vi "IO@SetPortName__Parameter.vi"(1 "ParamterIn":string) -> (0 "ParamterOut":string)   [LabVIEW 2020]
panel:
  in  "PortNameNew":string(combo)
  in  "PortSelect":string(combo)
  in  "Confirm":bool
  # "IO@SetPortName $IOOld,$IONew"
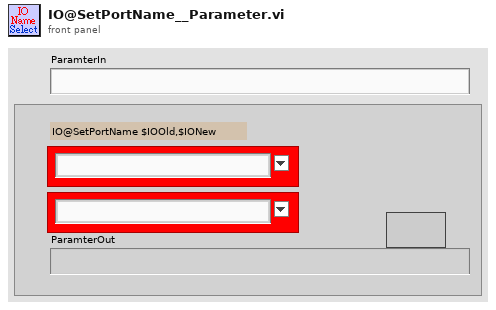
[diagram p1: front panel]
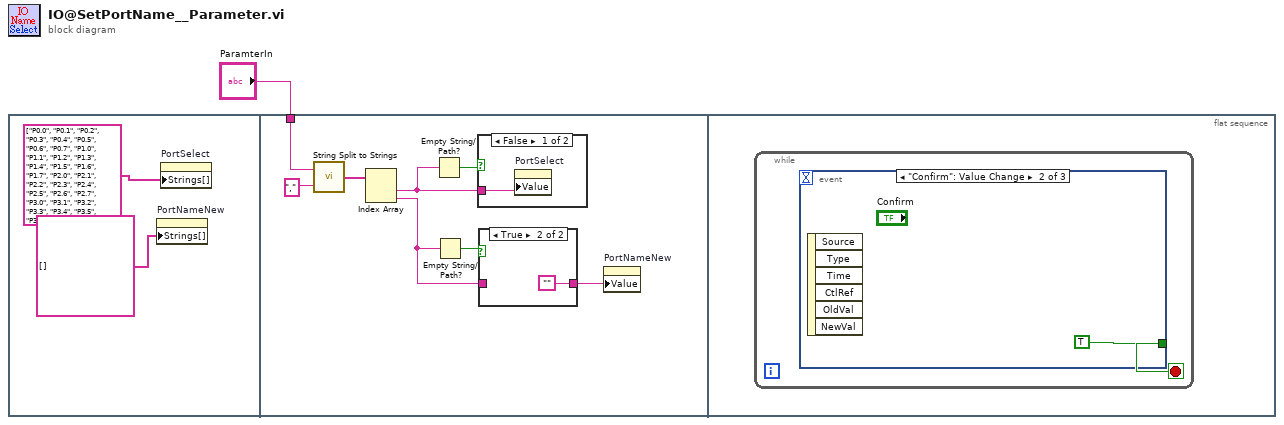
[diagram p0: block diagram]
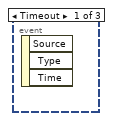
[diagram p4: hidden frame]
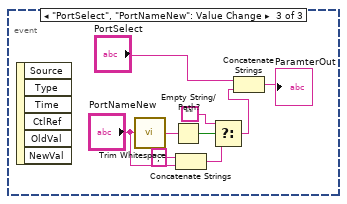
[diagram p5: hidden frame]
diagram:
  n1 = flat-sequence {
    tunnel: "ParamterIn" -> [w9]
    frame #0 {
      n2 = property on="PortNameNew" class="CmbBox"("Strings[]"=string[] [] ("Strings []")) -> ()  [unwired: 2 in, 2 out]
      n3 = property on="PortSelect" class="CmbBox"("Strings[]"=string[] ["P0.0", "P0.1", "P0.2", "P0.3", "P0.4", "P0.5", "P0.6", "P0.7", "P1.0", "P1.1", "P1.2", "P1.3", "P1.4", "P1.5", "P1.6", "P1.7", "P2.0", "P2.1", "P2.2", "P2.3", "P2.4", "P2.5", "P2.6", "P2.7", "P3.0", "P3.1", "P3.2", "P3.3", "P3.4", "P3.5", "P3.6", "P3.7", "P4.0", "P4.1", "P4.2", "P4.3", "P4.4", "P4.5", "P4.6", "P4.7", "P5.0", "P5.1", "P5.2", "P5.3", "P5.4", "P5.5", "P5.6", "P5.7", "P6.0", "P6.1", "P6.2", "P6.3", "P6.4", "P6.5", "P6.6", "P6.7", "P7.0", "P7.1", "P7.2", "P7.3", "P7.4", "P7.5", "P7.6", "P7.7", "P8.0", "P8.1", "P8.2", "P8.3", "P8.4", "P8.5", "P8.6", "P8.7", "P9.0", "P9.1", "P9.2", "P9.3", "P9.4", "P9.5", "P9.6", "P9.7", "P10.0", "P10.1", "P10.2", "P10.3", "P10.4", "P10.5", "P10.6", "P10.7", "P11.0", "P11.1", "P11.2", "P11.3", "P11.4", "P11.5", "P11.6", "P11.7", "P12.0", "P12.1", "P12.2", "P12.3", "P12.4", "P12.5", "P12.6", "P12.7", "P13.0", "P13.1", "P13.2", "P13.3", "P13.4", "P13.5", "P13.6", "P13.7", "P14.0", "P14.1", "P14.2", "P14.3", "P14.4", "P14.5", "P14.6", "P14.7", "P15.0", "P15.1", "P15.2", "P15.3", "P15.4", "P15.5", "P15.6", "P15.7", "P16.0", "P16.1", "P16.2", "P16.3", "P16.4", "P16.5", "P16.6", "P16.7", "P17.0", "P17.1", "P17.2", "P17.3", "P17.4", "P17.5", "P17.6", "P17.7", "P18.0", "P18.1", "P18.2", "P18.3", "P18.4", "P18.5", "P18.6", "P18.7", "P19.0", "P19.1", "P19.2", "P19.3", "P19.4", "P19.5", "P19.6", "P19.7", "P20.0", "P20.1", "P20.2", "P20.3", "P20.4", "P20.5", "P20.6", "P20.7", "P21.0", "P21.1", "P21.2", "P21.3", "P21.4", "P21.5", "P21.6", "P21.7", "P22.0", "P22.1", "P22.2", "P22.3", "P22.4", "P22.5", "P22.6", "P22.7", "P23.0", "P23.1", "P23.2", "P23.3", "P23.4", "P23.5", "P23.6", "P23.7", "P24.0", "P24.1", "P24.2", "P24.3", "P24.4", "P24.5", "P24.6", "P24.7", "P25.0", "P25.1", "P25.2", "P25.3", "P25.4", "P25.5", "P25.6", "P25.7", "P26.0", "P26.1", "P26.2", "P26.3", "P26.4", "P26.5", "P26.6", "P26.7", "P27.0", "P27.1", "P27.2", "P27.3", "P27.4", "P27.5", "P27.6", "P27.7", "P28.0", "P28.1", "P28.2", "P28.3", "P28.4", "P28.5", "P28.6", "P28.7", "P29.0", "P29.1", "P29.2", "P29.3", "P29.4", "P29.5", "P29.6", "P29.7", "P30.0", "P30.1", "P30.2", "P30.3", "P30.4", "P30.5", "P30.6", "P30.7", "P31.0", "P31.1", "P31.2", "P31.3", "P31.4", "P31.5", "P31.6", "P31.7", "P32.0", "P32.1", "P32.2", "P32.3", "P32.4", "P32.5", "P32.6", "P32.7", "P33.0", "P33.1", "P33.2", "P33.3", "P33.4", "P33.5", "P33.6", "P33.7", "P34.0", "P34.1", "P34.2", "P34.3", "P34.4", "P34.5", "P34.6", "P34.7", "P35.0", "P35.1", "P35.2", "P35.3", "P35.4", "P35.5", "P35.6", "P35.7", "P36.0", "P36.1", "P36.2", "P36.3", "P36.4", "P36.5", "P36.6", "P36.7", "P37.0", "P37.1", "P37.2", "P37.3", "P37.4", "P37.5", "P37.6", "P37.7", "P38.0", "P38.1", "P38.2", "P38.3", "P38.4", "P38.5", "P38.6", "P38.7", "P39.0", "P39.1", "P39.2", "P39.3", "P39.4", "P39.5", "P39.6", "P39.7", "P40.0", "P40.1", "P40.2", "P40.3", "P40.4", "P40.5", "P40.6", "P40.7", "P41.0", "P41.1", "P41.2", "P41.3", "P41.4", "P41.5", "P41.6", "P41.7", "P42.0", "P42.1", "P42.2", "P42.3", "P42.4", "P42.5", "P42.6", "P42.7", "P43.0", "P43.1", "P43.2", "P43.3", "P43.4", "P43.5", "P43.6", "P43.7", "P44.0", "P44.1", "P44.2", "P44.3", "P44.4", "P44.5", "P44.6", "P44.7", "P45.0", "P45.1", "P45.2", "P45.3", "P45.4", "P45.5", "P45.6", "P45.7", "P46.0", "P46.1", "P46.2", "P46.3", "P46.4", "P46.5", "P46.6", "P46.7", "P47.0", "P47.1", "P47.2", "P47.3", "P47.4", "P47.5", "P47.6", "P47.7", "P48.0", "P48.1", "P48.2", "P48.3", "P48.4", "P48.5", "P48.6", "P48.7", "P49.0", "P49.1", "P49.2", "P49.3", "P49.4", "P49.5", "P49.6", "P49.7", "P50.0", "P50.1", "P50.2", "P50.3", "P50.4", "P50.5", "P50.6", "P50.7", "P51.0", "P51.1", "P51.2", "P51.3", "P51.4", "P51.5", "P51.6", "P51.7", "P52.0", "P52.1", "P52.2", "P52.3", "P52.4", "P52.5", "P52.6", "P52.7", "P53.0", "P53.1", "P53.2", "P53.3", "P53.4", "P53.5", "P53.6", "P53.7", "P54.0", "P54.1", "P54.2", "P54.3", "P54.4", "P54.5", "P54.6", "P54.7", "P55.0", "P55.1", "P55.2", "P55.3", "P55.4", "P55.5", "P55.6", "P55.7", "P56.0", "P56.1", "P56.2", "P56.3", "P56.4", "P56.5", "P56.6", "P56.7", "P57.0", "P57.1", "P57.2", "P57.3", "P57.4", "P57.5", "P57.6", "P57.7", "P58.0", "P58.1", "P58.2", "P58.3", "P58.4", "P58.5", "P58.6", "P58.7", "P59.0", "P59.1", "P59.2", "P59.3", "P59.4", "P59.5", "P59.6", "P59.7", "P60.0", "P60.1", "P60.2", "P60.3", "P60.4", "P60.5", "P60.6", "P60.7", "P61.0", "P61.1", "P61.2", "P61.3", "P61.4", "P61.5", "P61.6", "P61.7", "P62.0", "P62.1", "P62.2", "P62.3", "P62.4", "P62.5", "P62.6", "P62.7", "P63.0", "P63.1", "P63.2", "P63.3", "P63.4", "P63.5", "P63.6", "P63.7"] ("Ports")) -> ()  [unwired: 2 in, 2 out]
    }
    frame #1 {
      n4 = call "String Split to Strings.vi"("search string/char (-)"=",", "String"=w9) -> ("Array"=w10:string[])
      n5 = Index Array(array=w10) -> (element #1=w7:string, element #2=w5:string)  [unwired: 2 in]
      n6 = Empty String/Path?(string/path=w7) -> (empty?=w8:bool)
      n7 = Empty String/Path?(string/path=w5) -> (empty?=w6:bool)
      n8 = case shown="False" w8 {
        tunnel: w7 -> [w14 _]
        frame False {
          n9 = property on="PortSelect" class="CmbBox"("Value"=w14) -> ()  [unwired: 2 in, 2 out]
        }
        frame True {
        }
      }
      n10 = case shown="True" w6 {
        tunnel: w5 -> [w12 _]
        tunnel: [w12 ""] -> w4
        frame False {
        }
        frame True {
        }
      }
      n11 = property on="PortNameNew" class="CmbBox"("Value"=w4) -> ()  [unwired: 2 in, 2 out]
    }
    frame #2 {
      n12 = while {
        stop <- w15 stop-if-true
        n13 = event shown="[1] \"Confirm\": Value Change" {
          selector: _ -> [_ _ _]
          dyn-events: _ -> [_ _ _]
          timeout: _ -> [_ _ _]
          tunnel: [_ TRUE _] -> w15
          event Timeout {
            n14 = event-data() -> ()  [unwired: 1 in, 3 out]
          }
          event "Confirm": Value Change {
            n15 = event-data() -> ()  [unwired: 1 in, 6 out]
          }
          event "PortSelect", "PortNameNew": Value Change {
            n16 = event-data() -> ()  [unwired: 1 in, 6 out]
            n17 = call <vilib>:"Trim Whitespace.vi"("string"="PortNameNew") -> ("trimmed string"=w23:string)  [unwired: 1 in]
            n18 = Empty String/Path?(string/path=w23) -> (empty?=w22:bool)
            n19 = Concatenate Strings("," ("string"), "PortNameNew") -> (w20:string)
            n20 = Select(t="", s=w22, f=w20) -> (s? t:f=w17:string)
            n21 = Concatenate Strings("PortSelect", w17) -> (→"ParamterOut":string)
          }
        }
      }
    }
  }
